vi "INST_PS_INIT_TURN_OFF_1.0.0.vi"(4 "Ouput(On:T)":bool, 8 "error in (no error)":errorcluster, 11 "VISA session":refnum<visa-resource-name>="GPIB0::10::INSTR") -> (0 "error out":errorcluster, 3 "dup VISA session":refnum<visa-resource-name>="GPIB0::10::INSTR")   [LabVIEW 2018]
doc: "This VI configures the power supply's voltage and current outputs. It sets the voltage and current parameters, in addition to setting which mode (immediate or triggered) the voltage and current is to function. This VI turns the output of the supply on and off. \n\nSupports E36xx, and 6634B"
panel:
  # "On\nOff"
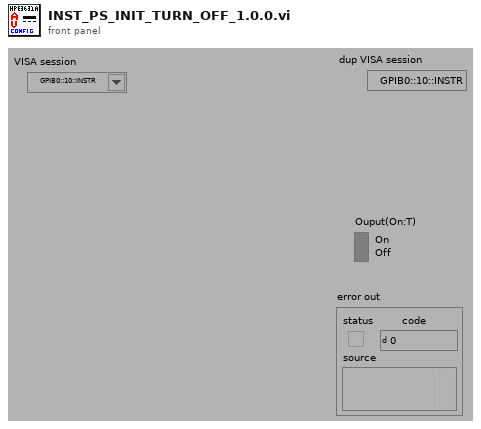
[diagram p1: front panel]
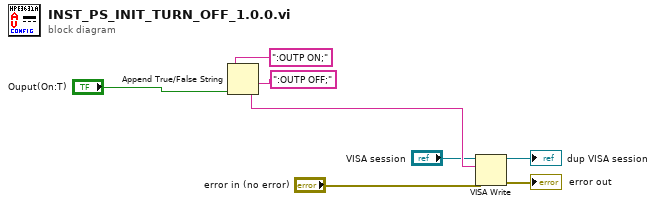
[diagram p0: block diagram]
diagram:
  n1 = Append True/False String(1:"Ouput(On:T)", 2:":OUTP OFF;", 3:":OUTP ON;") -> (0:w8:string)  [unwired: 1 in]
  n2 = VISA Write(VISA resource name="VISA session", write buffer=w8, error in (no error)="error in (no error)") -> (VISA resource name out=→"dup VISA session":refnum<visa-resource-name>, error out=→"error out":errorcluster)  [unwired: 1 out]
